vi "Flappy Tracker.vi"(8 "error in (no error)":errorcluster) -> (0 "error out":errorcluster)   [LabVIEW 2014]
uses:
  FlappyHeightPoint.ctl
  Globals.vi
panel:
  in  "FlappyHeightHistory":T1[](array[typedef])
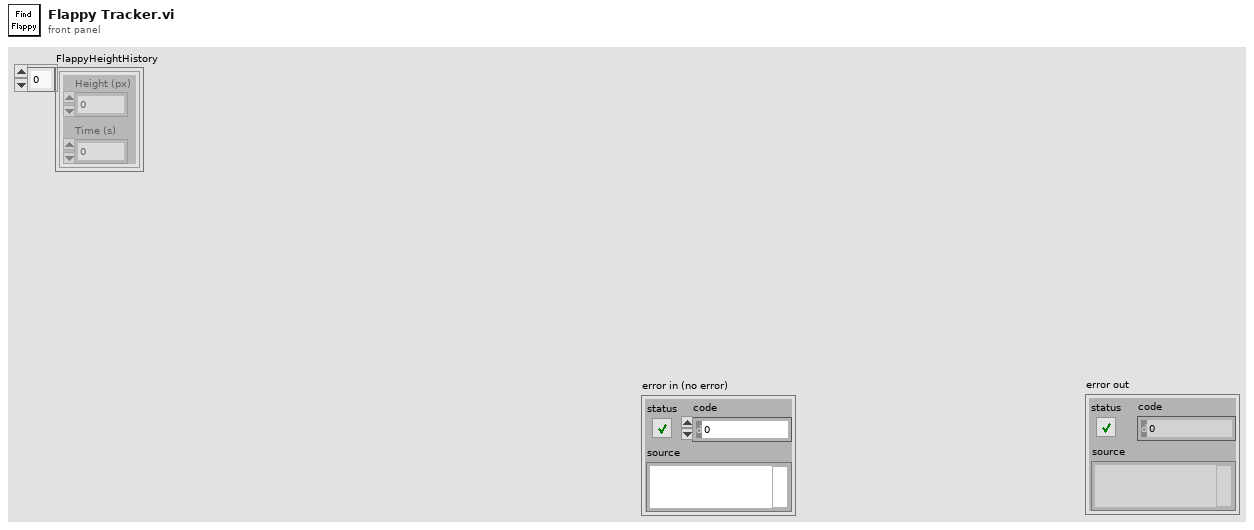
[diagram p1: front panel]
types:
  T1 = typedef "FlappyHeightPoint.ctl" = cluster{"Time (s)":dbl, "Height (px)":dbl}
  T2 = typedef "IMAQ Image.ctl" = refnum<image>
  T3 = typedef "ImageCluster.ctl" = cluster{"Screenshot":T2, "Time (s)":dbl}
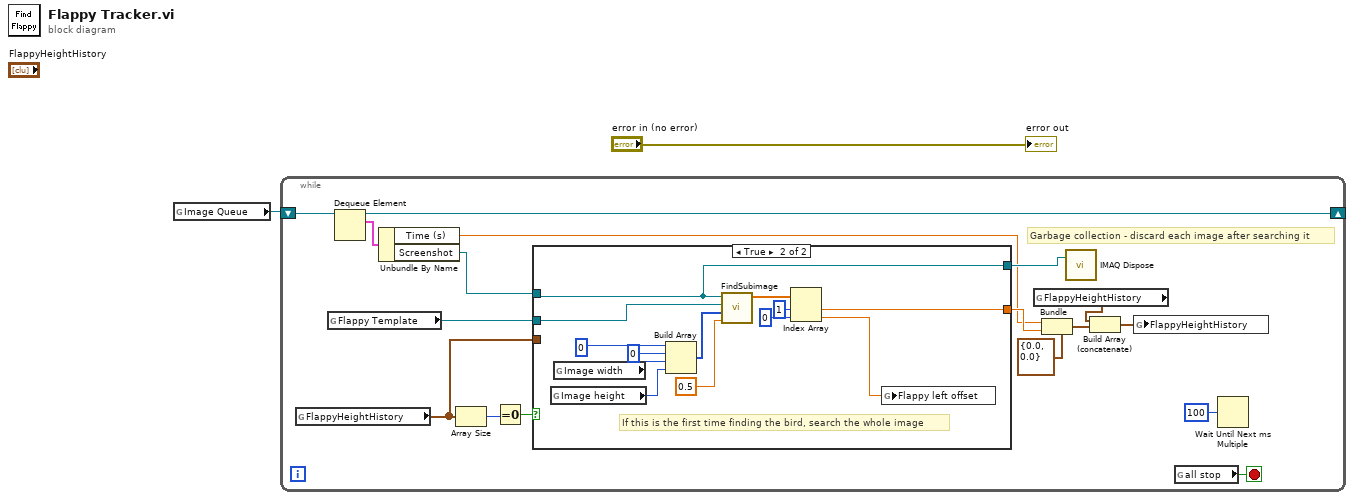
[diagram p0: block diagram]
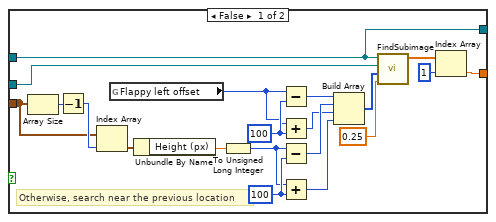
[diagram p2: hidden frame]
diagram:
  n1 = global read "Globals.vi" "Image Queue"() -> (w2:refnum<queue>)
  n2 = while {
    shift-right: [w16] -> _
    shift-left: w2 -> [w17]
    stop <- w9 stop-if-true
    # "Garbage collection - discard each image after searching it"
    n3 = global read "Globals.vi" "FlappyHeightHistory"() -> (w6:T1[])
    n4 = global read "Globals.vi" "Flappy Template"() -> (w11:T2)
    n5 = Dequeue Element(queue=w17) -> (queue out=w16:refnum<queue>, element=w15:T3)  [unwired: 2 in, 2 out]
    n6 = Unbundle By Name(w15) -> ("Time (s)"=w4:dbl, "Screenshot"=w14:T2)
    n7 = Array Size(array=w6) -> (size(s)=w19:i32)
    n8 = Equal To 0?(x=w19) -> (x = 0?=w18:bool)
    n9 = case shown="True" w18 {
      tunnel: w11 -> [w36 w52]
      tunnel: [w38 w49] -> w5
      tunnel: w14 -> [w22 w44]
      tunnel: w6 -> [w29 _]
      tunnel: [w22 w44] -> w10
      frame False {
        w28 = u32 100 ("y")
        w33 = u32 100 ("y")
        # "Otherwise, search near the previous location"
        n10 = Array Size(array=w29) -> (size(s)=w35:i32)
        n11 = Decrement(x=w35) -> (x-1=w34:i32)
        n12 = Index Array(array=w29, index=w34) -> (element=w25:T1)
        n13 = global read "Globals.vi" "Flappy left offset"() -> (w23:u32)
        n14 = Unbundle By Name(w25) -> ("Height (px)"=w20:dbl)
        n15 = To Unsigned Long Integer(number=w20) -> (unsigned 32bit integer=w24:u32)
        n16 = Subtract(x=w23, y=w28) -> (x-y=w27:u32)
        n17 = Add(x=w23, y=w28) -> (x+y=w26:u32)
        n18 = Subtract(x=w24, y=w33) -> (x-y=w32:u32)
        n19 = Add(x=w24, y=w33) -> (x+y=w31:u32)
        n20 = Build Array(w27, w32, w26, w31) -> (w30:u32[])
        n21 = call "FindSubimage.vi"("Scale factor (1)"=0.25, "ROI (left top right bottom)"=w30, "RGB Template"=w36, "RGB Image"=w22) -> ("Locations (left, top)"=w37:dbl[])  [unwired: 7 in]
        n22 = Index Array(array=w37, index=1) -> (element=w38:dbl)
      }
      frame True {
        # "If this is the first time finding the bird, search the whole image"
        n23 = global read "Globals.vi" "Image height"() -> (w45:u32)
        n24 = global read "Globals.vi" "Image width"() -> (w43:u32)
        n25 = Build Array(0 ("element"), 0 ("element"), w43, w45) -> (w47:u32[])
        n26 = call "FindSubimage.vi"("Scale factor (1)"=0.5, "ROI (left top right bottom)"=w47, "RGB Template"=w52, "RGB Image"=w44) -> ("Locations (left, top)"=w51:dbl[])  [unwired: 7 in]
        n27 = Index Array(array=w51, index #1=1 ("index"), index #2=0 ("index")) -> (element #1=w49:dbl, element #2=w40:dbl)
        n28 = global write "Globals.vi" "Flappy left offset"(w40) -> ()
      }
    }
    n29 = global read "Globals.vi" "FlappyHeightHistory"() -> (w7:T1[])
    n30 = Bundle(cluster=T1 {"Time (s)"=0.0, "Height (px)"=0.0}, "Time (s)"=w4, "Height (px)"=w5) -> (w12:T1)
    n31 = call "IMAQ Dispose"("Image"=w10) -> ()  [unwired: 5 in, 1 out]
    n32 = Build Array (concatenate)(w7, w12) -> (w8:T1[])
    n33 = global write "Globals.vi" "FlappyHeightHistory"(w8) -> ()
    n34 = global read "Globals.vi" "all stop"() -> (w9:bool)
    n35 = Wait Until Next ms Multiple(millisecond multiple=u32 100) -> ()  [unwired: 1 out]
  }
  "error out" <- "error in (no error)"
